vi "Compound.vi"(8 "error in (no error)":errorcluster, 10 "Time Stamp":timestamp, 11 "IInterest in":refnum<class "IInterest.lvclass">) -> (0 "error out":errorcluster, 3 "IInterest out":refnum<class "IInterest.lvclass">)   [LabVIEW 2020, in "IInterest.lvclass"]
uses:
  IInterest.lvclass
panel:
  out "Balance":dbl
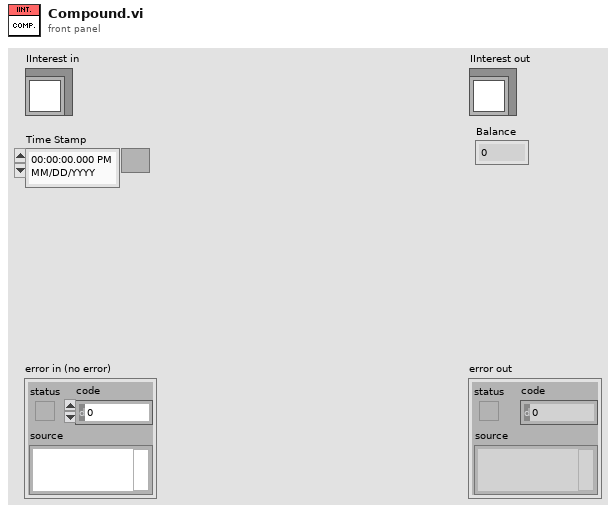
[diagram p1: front panel]
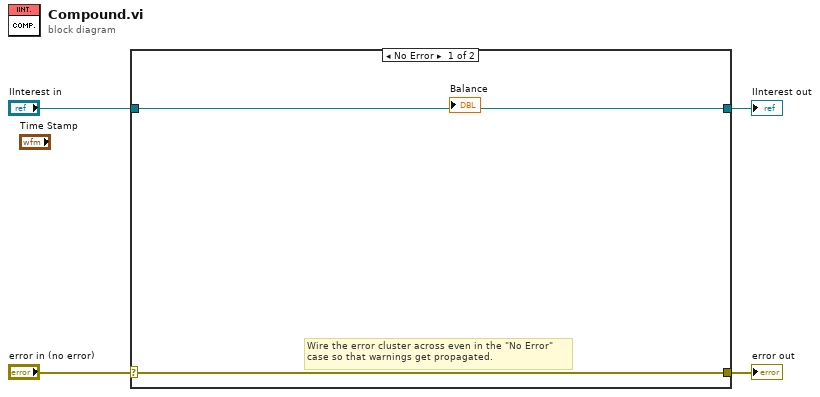
[diagram p0: block diagram]
diagram:
  n1 = case shown="No Error" "error in (no error)" {
    selector: "error in (no error)" -> [w5 w8]
    tunnel: [w5 w8] -> w3
    tunnel: [w6 w7] -> w1
    tunnel: "IInterest in" -> [w6 w7]
    frame No Error {
      # "Wire the error cluster across even in the \"No Error\"\ncase so that warnings get propagated."
    }
    frame Error {
    }
  }
  "error out" <- w3
  "IInterest out" <- w1
